vi "Parse Serial Data.vi"(5 "Serial String":string, 11 "error in":errorcluster) -> (4 "Pressure":dbl, 6 "Temp1":dbl, 8 "Temp2":dbl, 10 "Temp3":dbl, 15 "error out":errorcluster)   [LabVIEW 2021]
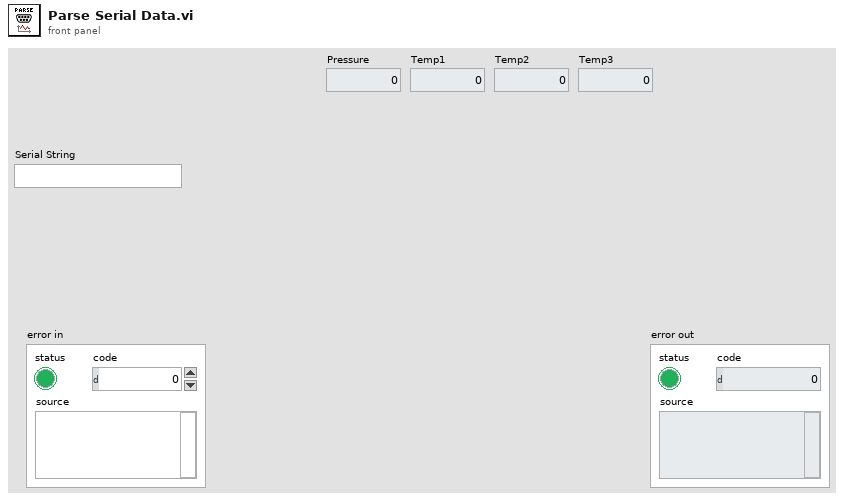
[diagram p1: front panel]
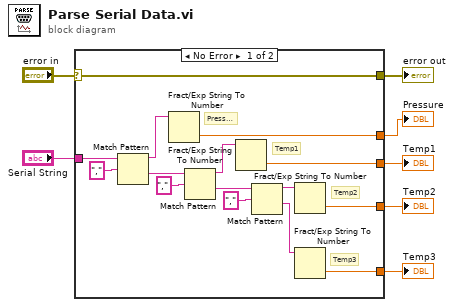
[diagram p0: block diagram]
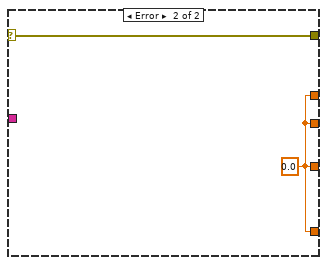
[diagram p2: hidden frame]
diagram:
  n1 = case shown="No Error" "error in" {
    selector: "error in" -> [w22 w24]
    tunnel: [w22 w24] -> w6
    tunnel: "Serial String" -> [w21 _]
    tunnel: [w11 w23] -> w5
    tunnel: [w10 w23] -> w4
    tunnel: [w9 w23] -> w3
    tunnel: [w8 w23] -> w2
    frame No Error {
      # "Temp3"
      # "Temp2"
      # "Temp1"
      # "Pressure"
      n2 = Match Pattern(string=w21, regular expression=",") -> (before substring=w19:string, after substring=w18:string)  [unwired: 1 in, 2 out]
      n3 = Fract/Exp String To Number(string=w19) -> (number=w11:dbl)  [unwired: 3 in, 1 out]
      n4 = Match Pattern(string=w18, regular expression=",") -> (before substring=w16:string, after substring=w15:string)  [unwired: 1 in, 2 out]
      n5 = Fract/Exp String To Number(string=w16) -> (number=w10:dbl)  [unwired: 3 in, 1 out]
      n6 = Match Pattern(string=w15, regular expression=",") -> (before substring=w13:string, after substring=w12:string)  [unwired: 1 in, 2 out]
      n7 = Fract/Exp String To Number(string=w13) -> (number=w9:dbl)  [unwired: 3 in, 1 out]
      n8 = Fract/Exp String To Number(string=w12) -> (number=w8:dbl)  [unwired: 3 in, 1 out]
    }
    frame Error {
      w23 = 0.0
    }
  }
  "error out" <- w6
  "Pressure" <- w5
  "Temp1" <- w4
  "Temp2" <- w3
  "Temp3" <- w2
